vi "SbigDecodeBCD.vi"(1 "Format":string, 2 "Array of U16":u16[](array[numeric])) -> (7 "nombre":dbl format="%.2f")   [LabVIEW 2009]
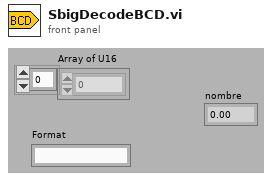
[diagram p1: front panel]
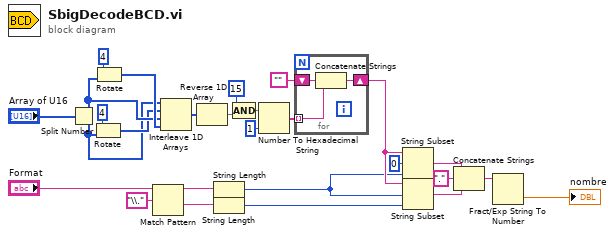
[diagram p0: block diagram]
diagram:
  n1 = Split Number(x="Array of U16") -> (hi(x)=w3:u8[], lo(x)=w1:u8[])
  n2 = Rotate(1:w1, 2:i16 4 ("y")) -> (0:w2:u8[])
  n3 = Rotate(1:w3, 2:i16 4 ("y")) -> (0:w4:u8[])
  n4 = Match Pattern(string="Format", regular expression="\\." ("expression")) -> (before substring=w19:string, after substring=w18:string)  [unwired: 3 out]
  n5 = Interleave 1D Arrays(w1, w2, w3, w4) -> (w6:u8[])
  n6 = Reverse 1D Array(array=w6) -> (reversed array=w5:u8[])
  n7 = String Length(string=w19) -> (length=w12:i32)
  n8 = String Length(string=w18) -> (length=w13:i32)
  n9 = Compound Arithmetic op=AND(u8 15 ("Entrée"), w5) -> (w27:u8[])
  n10 = Number To Hexadecimal String(1:i16 1 ("largeur (-)"), 2:w27) -> (0:w17:string[])
  n11 = for {
    tunnel: w17 -> [w29] mode=indexing
    shift-right: [w30] -> w15
    shift-left: "" -> [w28]
    n12 = Concatenate Strings(w28, w29) -> (w30:string)
  }
  n13 = String Subset(string=w15, offset (0)=0, length (rest)=w12) -> (substring=w11:string)
  n14 = String Subset(string=w15, offset (0)=w12, length (rest)=w13) -> (substring=w10:string)
  n15 = Concatenate Strings(w11, ".", w10) -> (w8:string)
  n16 = Fract/Exp String To Number(string=w8) -> (number=→"nombre":dbl)  [unwired: 4 out]
